vi "Application to add 2 numbers.vi"() -> ()   [LabVIEW 2022 SP3]
panel:
  in  "Boolean":bool
  out "Numeric 3":dbl
  in  "Numeric 2":dbl
  in  "Numeric":dbl
  # "Example: Building an application to calculate the product of two numbers"
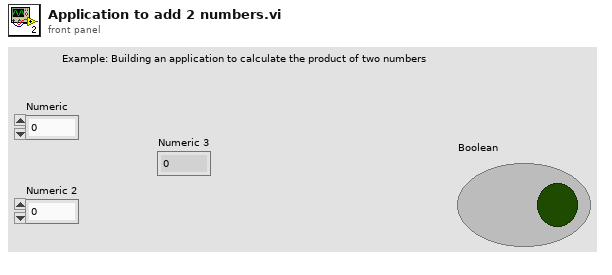
[diagram p1: front panel]
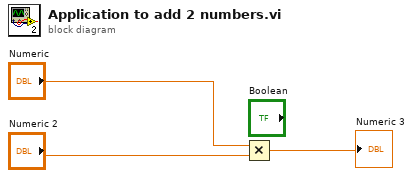
[diagram p0: block diagram]
diagram:
  n1 = Multiply(x="Numeric", y="Numeric 2") -> (x*y=→"Numeric 3":dbl)
